vi "0805_Visão_de_máquina.vi"() -> ()   [LabVIEW 2017]
uses:
  <vilib>/userdefined/High Color/IMAQdx.ctl
  <vilib>/vision/driver/IMAQdx.llb/IMAQdx Acquisition Mode.ctl
  <vilib>/vision/driver/IMAQdx.llb/IMAQdx Buffer Number Mode.ctl
  <vilib>/vision/Classification.llb/IMAQ Classifier Read Options.ctl
  <vilib>/vision/driver/NI_Vision_Acquisition_Software.lvlib
  <vilib>/vision/NI_Vision_Development_Module.lvlib
panel:
  out "seletou_detectou":bool
  in  "file (use dialog)":path
  in  "Comunicação de dados":bool
  out "concatenated string 2":string
  out "concatenated string":string
  out "Boolean":bool
  out "Parar_esteira":bool
  out "aux":bool
  out "normal":u32
  out "parou":u32
  out "detectou":u32
  out "Detectou":bool
  out "reconheceu":bool
  out "bool_parou":bool
  out "bool_normal":bool
  out "bool_detectou":bool
  out "reconhecendo":bool
  out "Stop 3":bool
  out "seletor":enum16{"normal", "detectou", "parou"}(ring)=enum."detectou"
  in  "enum":enum16{"normal", "detectou", "parou"}(ring)=enum."detectou"
  out "x .and. y?":bool
  in  "dimensão_x_ROI_esteira":sgl=30.0
  in  "dimensão_y_ROI_esteira":sgl=30.0
  in  "posicao_y_ROI_esteira":sgl
  in  "posicao_x_ROI_esteira":sgl
  out "Local destino":T1(ring)
  in  "Tab Control":T2(tab)
  in  "Cluster A":T3
  in  "Cluster B":T3
  in  "Cluster C":T3
  in  "QRCode":bool
  out "Table":string[][](table)
  in  "Stop 2":bool
  in  "Stop 1":bool
  out "Imagem Original":T4(plugin-control)
  in  "Câmera":T5="cam1"
  out "XY Graph 2":cluster{"X":dbl, "Y":dbl}[](graph)
  # "ROTINA DE VISÃO COMPUTACIONAL"
  # "HISTÓRICO DE RECONHECIMENTO"
  # "DEFINI敲O DA ROI DA ESTEIRA"
  # "IMAGEM OBTIDA PELA CÂMERA"
  # "POSI敲O X"
  # "-100"
  # "POSI敲O Y"
  # "-230"
  # "DIMENSÃO X"
  # "80"
  # "DIMENSÃO Y"
  # "250"
  # "DEFINI敲O DOS LOCAIS DE DESTINO\nDA MANIPULA敲O"
  # "LOCAL DE DESTINO"
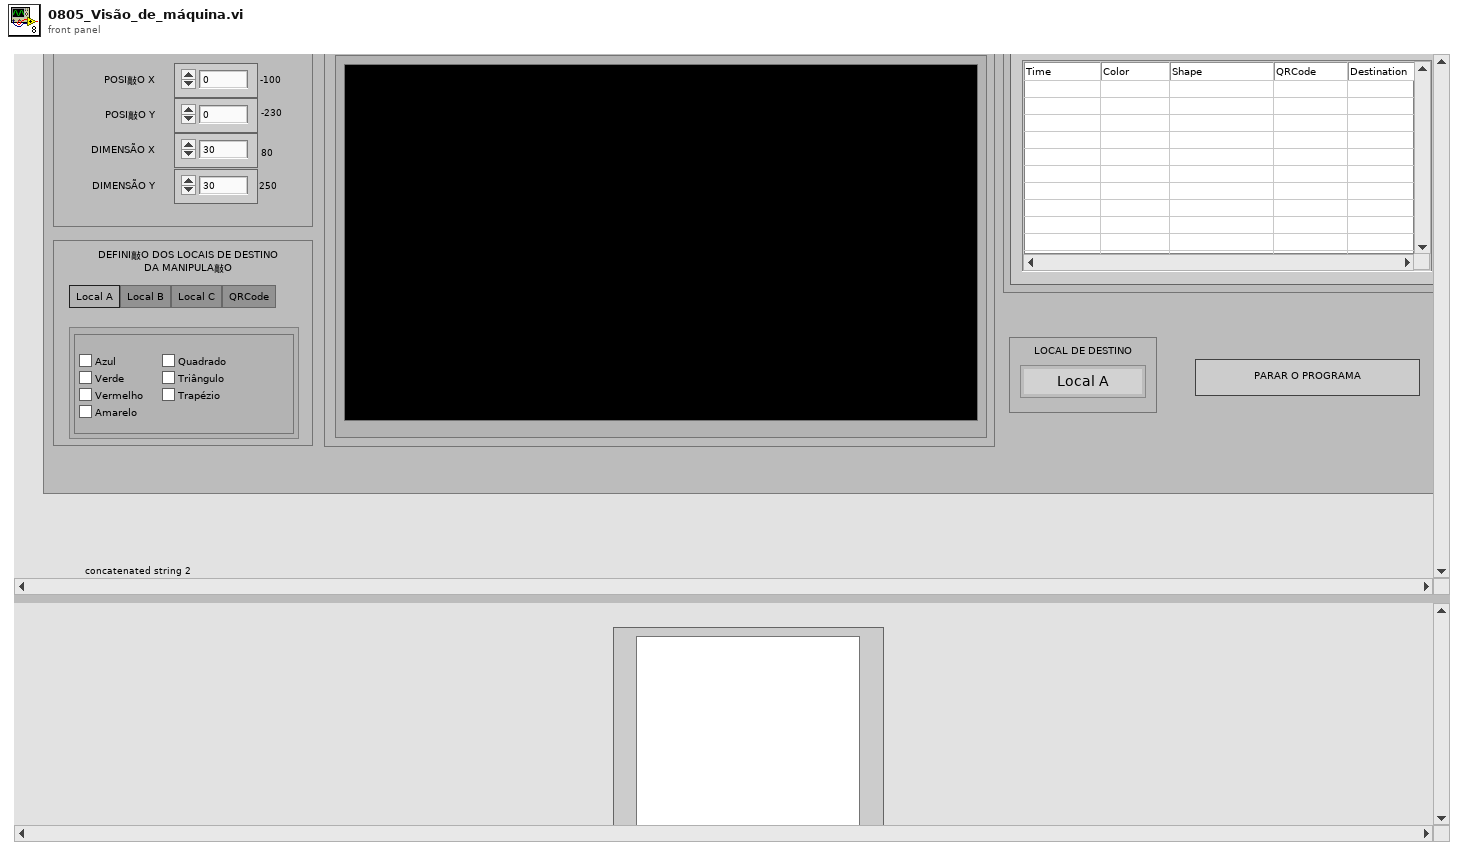
[diagram p1: front panel]
types:
  T1 = enum16{"Local A", "Local B", "Local C", "Discard"}
  T2 = enum32{"Local A", "Local B", "Local C", "QRCode"}
  T3 = cluster{"Azul":bool, "Verde":bool, "Vermelho":bool, "Amarelo":bool, "Quadrado":bool, "Triângulo":bool, "Trapézio":bool}
  T4 = typedef "IMAQ Image.ctl" = refnum<image>
  T5 = typedef "IMAQdx.ctl" = refnum<k21>
  T6 = typedef "NI_Vision_Acquisition_Software.lvlib/IMAQdx Acquisition Mode.ctl" = enum32{"One Shot", "Continuous"}
  T7 = typedef "NI_Vision_Acquisition_Software.lvlib/IMAQdx Buffer Number Mode.ctl" = enum32{"Next", "Last", "Buffer Number", "Every", "Last New"}
  T8 = cluster{"Global Rectangle":i32[], "Contours":cluster{"Contour Type":u32, "ROI Type":u32, "Points":i32[]}[]}
  T9 = typedef "ROI Descriptor" = cluster{"Global Rectangle":i32[], "Contours":cluster{"ID":enum32{"External", "Internal"}, "Type":u32, "Coordinates":i32[]}[]}
  T10 = typedef "IMAQ Classifier Read Options.ctl" = i32
  T11 = typedef "IMAQ Classifier Session.ctl" = refnum<k1>
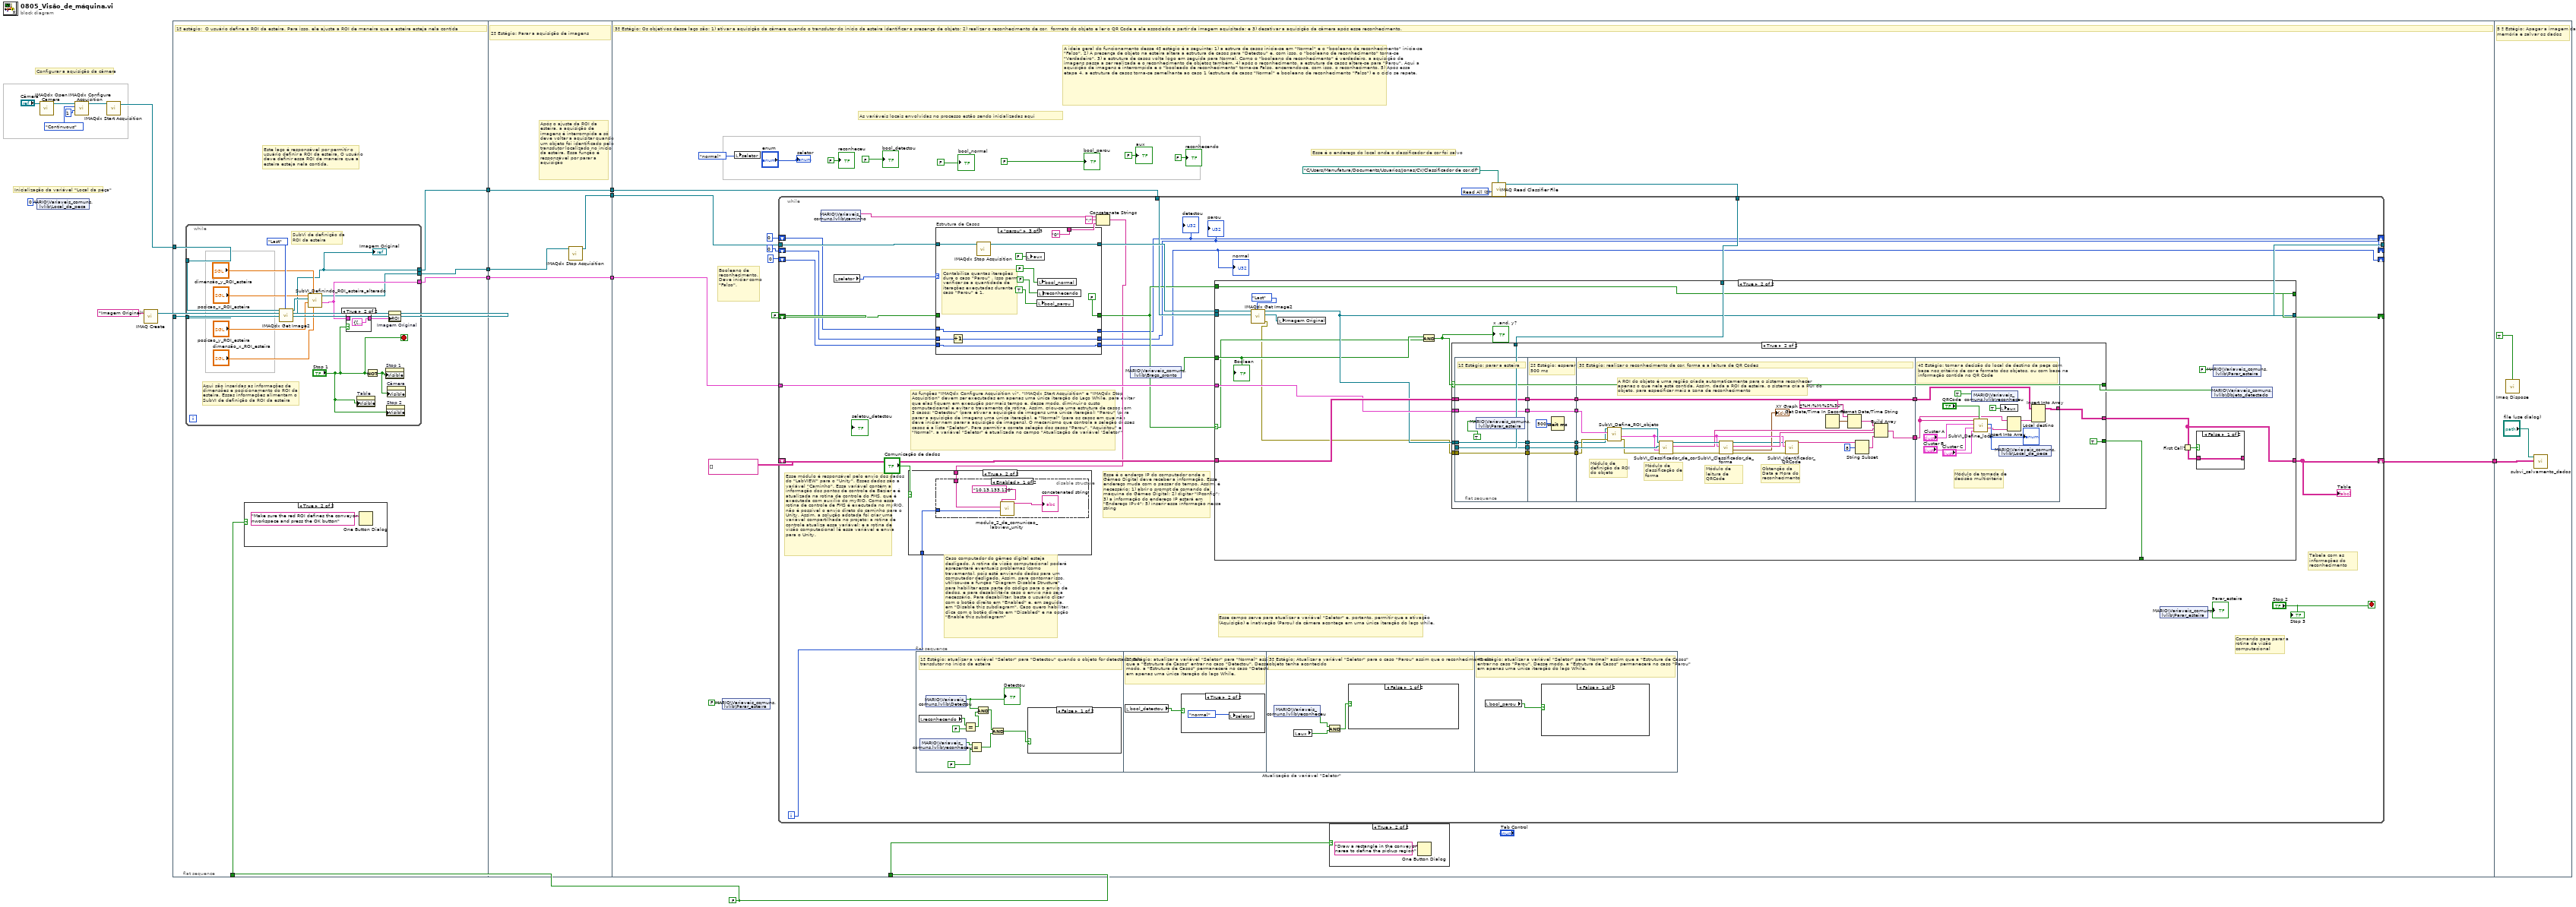
[diagram p0: block diagram]
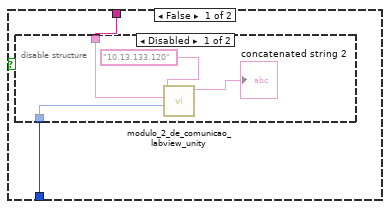
[diagram p4: hidden frame]
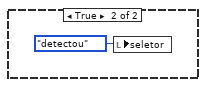
[diagram p7: hidden frame]
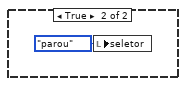
[diagram p9: hidden frame]
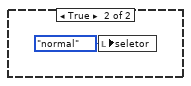
[diagram p10: hidden frame]
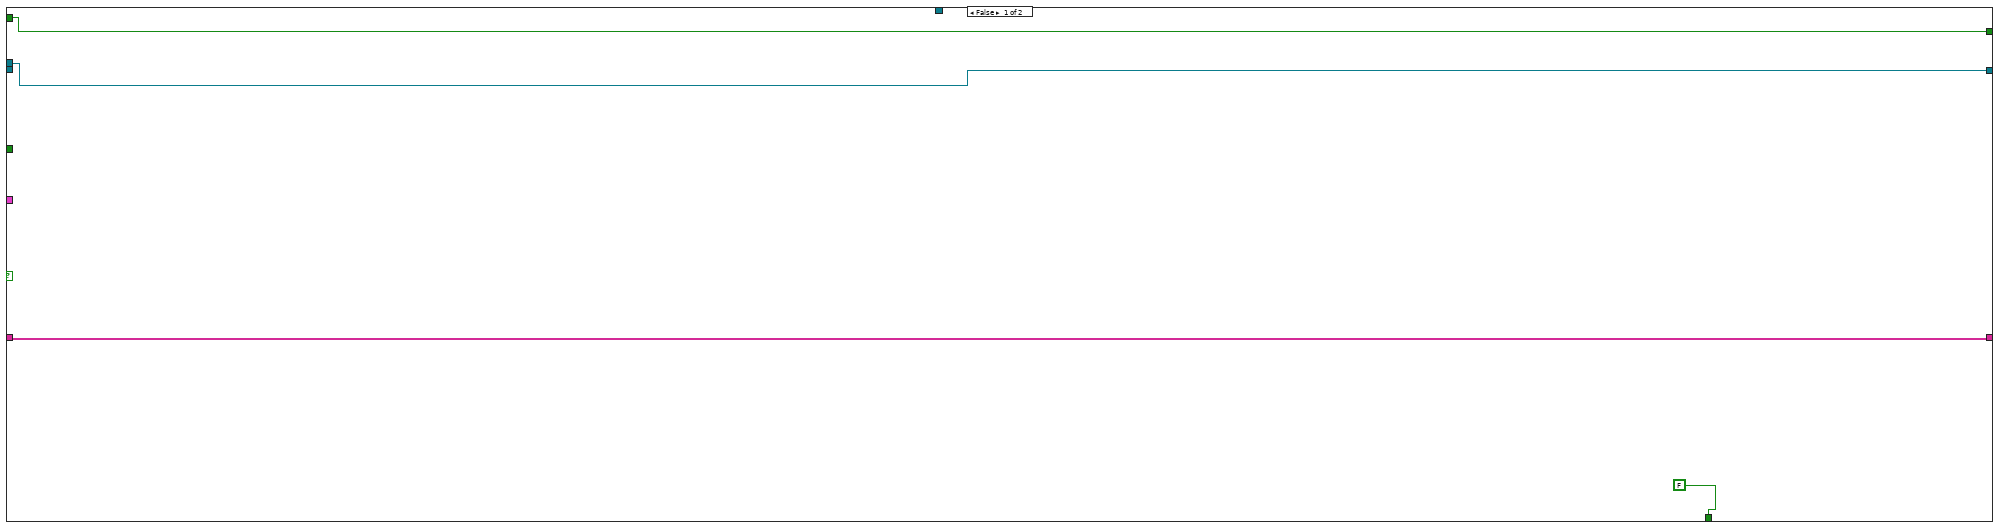
[diagram p11: hidden frame]
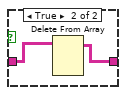
[diagram p12: hidden frame]
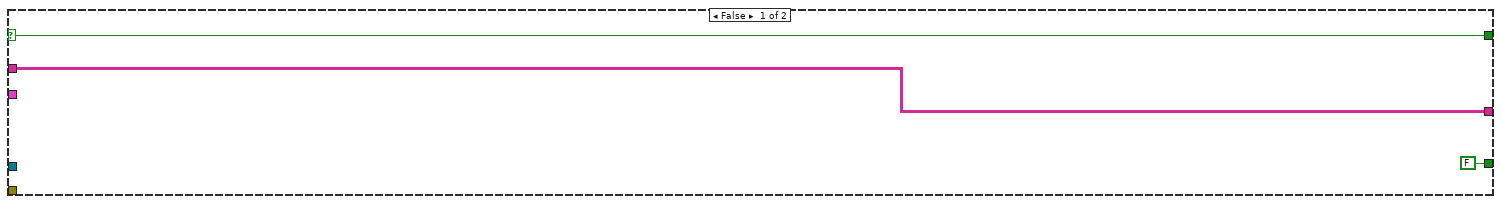
[diagram p13: hidden frame]
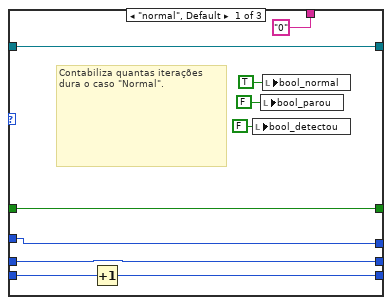
[diagram p14: hidden frame]
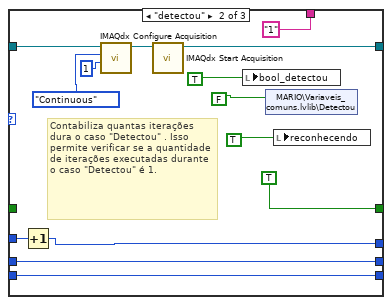
[diagram p15: hidden frame]
diagram:
  w10 = FALSE
  # "Inicialização da variável \"Local da peça\""
  # "Configurar a aquisição da câmera"
  n1 = shared-variable "MARIO\\Variaveis_comuns.lvlib\\Local_da_peca"(i8 0 ("Local_da_peca")) -> ()  [unwired: 1 in, 1 out]
  n2 = call <vilib>:"IMAQdx Open Camera.vi"("Session In"="Câmera") -> ("Session Out"=w17:T5)  [unwired: 9 in, 1 out]
  n3 = call <vilib>:"IMAQdx Configure Acquisition.vi"("Number of Buffers"=u32 1, "Continuous?"=IMAQdx_Acquisition_Mode."Continuous", "Session In"=w17) -> ("Session Out"=w16:T5)  [unwired: 7 in, 1 out]
  n4 = call <vilib>:"IMAQdx Start Acquisition.vi"("Session In"=w16) -> ("Session Out"=w7:T5)  [unwired: 9 in, 1 out]
  n5 = call "IMAQ Create"("Image Name"="Imagem Original") -> ("New Image"=w11:T4)  [unwired: 4 in, 1 out]
  n6 = flat-sequence {
    tunnel: w7 -> [w23]
    tunnel: w11 -> [w22]
    tunnel: [w21] -> w4
    tunnel: [w20] -> w3
    tunnel: [w19] -> w2
    tunnel: w10 -> [w18]
    tunnel: w4 -> [w43]
    tunnel: w3 -> [w44]
    tunnel: [w44] -> w9
    tunnel: [w42] -> w8
    tunnel: w2 -> [w42]
    tunnel: [w41] -> w6
    tunnel: w9 -> [w62]
    tunnel: w10 -> [w66]
    tunnel: w8 -> [w59]
    tunnel: w6 -> [w57]
    tunnel: [w45] -> w1
    tunnel: w1 -> [w256]
    frame #0 {
      # "Este laço é responsável por permitir o usuário definir a ROI da esteira. O usuário deve definir essa ROI de maneira que a esteira esteja nela contida."
      # "1º estágio:  O usuário define a ROI da esteira. Para isso, ele ajusta a ROI de maneira que a esteira esteja nela contida"
      n7 = while {
        tunnel: w23 -> [w37]
        tunnel: w22 -> [w36]
        tunnel: [w26] -> w21
        tunnel: [w27] -> w20
        tunnel: [w25] -> w19
        stop <- "Stop 1" stop-if-true
        # "SubVi de definição da ROI da esteira"
        # "Aqui são inseridas as informações de dimensões e posicionamento do ROI da esteira. Essas informações alimentam o SubVI de definição da ROI da esteira"
        n8 = call <vilib>:"IMAQdx Get Image2.vi"("Buffer Number Mode (Next)"=IMAQdx_Buffer_Number_Mode."Last", "Image In"=w36, "Session In"=w37) -> ("Image Out"=w25:T4, "Session Out"=w28:T5)  [unwired: 5 in, 2 out]
        "Imagem Original" <- w25
        n9 = call "SubVI_Definindo_ROI_esteira_alterado.vi"("largura_y"="dimensão_x_ROI_esteira", "largura_x"="dimensão_y_ROI_esteira", "ofset y"="posicao_y_ROI_esteira", "Session in"=w28, "ofset x"="posicao_x_ROI_esteira") -> ("ROI Descriptor"=w27:T9, "Session Out"=w26:T5)  [unwired: 4 in, 1 out]
        n10 = case shown="True" "Stop 1" {
          tunnel: w27 -> [w39 _]
          tunnel: [w39 T8 {"Global Rectangle"=[0, 0, 1, 1], "Contours"=[{"Contour Type"=0, "ROI Type"=1, "Points"=[0, 0]}]} ("ROI")] -> w35
          frame False {
          }
          frame True {
          }
        }
        n11 = property on="Table" class="Tbl (strict)"("Visible"="Stop 1") -> ()  [unwired: 2 in, 2 out]
        n12 = Not(x="Stop 1") -> (.not. x?=w34:bool)
        n13 = property on="Stop 1" class="Bool"("Visible"=w34) -> ()  [unwired: 2 in, 2 out]
        n14 = property on="Stop 2" class="Bool"("Visible"="Stop 1") -> ()  [unwired: 2 in, 2 out]
        n15 = property on="Câmera" class="IMAQdx (strict)"("Visible"=w34) -> ()  [unwired: 2 in, 2 out]
        n16 = property on="Imagem Original" class="ImageControl"("ROI"=w35) -> ()  [unwired: 2 in, 2 out]
      }
      n17 = case shown="True" w18 {
        frame False {
        }
        frame True {
          n18 = One Button Dialog(message="Make sure the red ROI defines the conveyor \nworkspace and press the OK button") -> ()  [unwired: 1 in, 1 out]
        }
      }
    }
    frame #1 {
      # "Após o ajuste da ROI da esteira, a aquisição de imagens é interrompida e só deve voltar a aquisitar quando um objeto foi identificado pelo transdutor localizado no início da esteira. Essa função é responsável por parar a aquisição"
      # "2º Estágio: Parar a aquisição de imagens"
      n19 = call <vilib>:"IMAQdx Stop Acquisition.vi"("Session In"=w43) -> ("Session Out"=w41:T5)  [unwired: 9 in, 1 out]
    }
    frame #2 {
      w65 = T10 0 items=["Read All", "Add Samples, Do Not Change Options", "Read Options, Do Not Add Samples"] ("Read Options")
      # "Esse é o endereço do local onde o classificador de cor foi salvo"
      # "A ideia geral do funcionamento desse 4º estágio é a seguinte: 1) a estrura de casos inicia-se em \"Normal\" e o \"booleano de reconhecimento\" inicia-se \"Falso\". 2) A presença de objeto na esteira altera a estrutura de casos para \"Detectou\" e, com isso, o \"booleano de reconhecimento\" torna-se \"Verdadeiro\". 3) a estrutura de casos volta logo em seguida para Normal. Como o \"booleano de reconhecimento\" é verdadeiro, a aquisição de imagens passa a ser realizada e o reconhecimento de objetos também. 4) após o reconhecimento, a estrutura de casos altera-se para \"Parou\". Aqui a aquisição de imagens é interrompida e o \"booleado de reconhecimento\" torna-se Falso, encerrando-se, com isso, o reconhecimento. 5) Após essa etapa 4, a estrutura de casos torna-se semelhante ao caso 1 (estrutura de casos \"Normal\" e booleano de reconhecimento \"Falso\") e o ciclo se repete."
      # "As variáveis locais envolvidas no processo estão sendo inicializadas aqui"
      # "Booleano de reconhecimento. Deve iniciar como \"Falso\"."
      # "3º Estágio: Os objetivos desse laço são: 1) ativar a aquisição da câmera quando o transdutor do início da esteira identificar a presença de objeto; 2) realizar o reconhecimento de cor,  formato do objeto e ler o QR Code a ele associado a partir da imagem aquisitada; e 3) desativar a aquisição da câmera após esse reconhecimento."
      n20 = shared-variable "MARIO\\Variaveis_comuns.lvlib\\Parar_esteira"(FALSE ("Parar_esteira")) -> ()  [unwired: 1 in, 1 out]
      n21 = local write "seletor"(enum16{"normal", "detectou", "parou"}."normal") -> ()
      n22 = case shown="True" w66 {
        frame False {
        }
        frame True {
          n23 = One Button Dialog(message="Draw a rectangle in the conveyor\narea to define the pickup region") -> ()  [unwired: 1 in, 1 out]
        }
      }
      n24 = call "IMAQ Read Classifier File"("File Path"=path "C:/Users/Manufatura/Documents/Usuarios/Jonas/CV/Classificador de cor.clf", "Read Options"=w65) -> ("Classifier Session"=w64:T11)  [unwired: 2 in, 7 out]
      n25 = while {
        tunnel: w62 -> [w92]
        tunnel: w64 -> [w93]
        shift-right: [w73] -> w45
        shift-left: string[][] [] ("Table") -> [w74]
        tunnel: w59 -> [w90]
        shift-right: [w87] -> _
        shift-left: FALSE -> [w89]
        tunnel: w57 -> [w85]
        tunnel: [w86] -> _
        shift-right: [w81] -> _
        shift-left: u32 0 ("Number of Buffers") -> [w78]
        shift-right: [w80] -> _
        shift-left: u32 0 ("Number of Buffers") -> [w77]
        shift-right: [w79] -> _
        shift-left: u32 0 ("Number of Buffers") -> [w76]
        i -> [w68]
        stop <- "Stop 2" stop-if-true
        # "Tabela com as informações do reconhecimento"
        # "Comando para parar a rotina de visão computacional"
        # "Esse campo serve para atualizar a variável \"Seletor\" e, portanto, permitir que a ativação (Aquisição) e inativação (Parou) da câmera aconteça em uma única iteração do laço while."
        # "Esse é o enderço IP do computador onde o Gêmeo Digital deve receber a informação. Esse endereço muda com o passar do tempo. Assim, é necessário: 1) abrir o prompt de comando da máquina do Gêmeo Digital; 2) digitar \"IPconfig\"; 3) a informação do endereço IP estará em \"Endereço IPv4\"; 5) inserir essa informação nessa string"
        # "Caso computador do gêmeo digital esteja desligado, A rotina de visão computacional poderá apresentará eventuais problemas (como travamento), pois está enviando dados para um computador desligado. Assim, para contornar isso, utilizou-se a função \"Diagram Disable Structure\", para habilitar essa parte do código para o envio de dados, e para desabilitá-la caso o envio não seja necessário. Para desabilitar, basta o usuário clicar com o botão direito em \"Enabled\" e, em seguida, em \"Disable this subdiagram\". Caso quero habilitar, clica com o botão direito em \"Disabled\" e na opção \"Enable this subdiagram\""
        # "Esse módulo é responsável pelo envio dos dados do \"LabVIEW\" para o \"Unity\". Esses dados são a variável \"Caminho\". Essa variável contém a informação dos pontos de controle de Bézier e é atualizada na rotina de controle do FMS, que é executada com auxílio do myRIO. Como essa rotina de controle de FMS é executada no myRIO, não é possível o envio direto do caminho para o Unity. Assim, a solução adotada foi criar uma  variável compartilhada no projeto: a rotina de controle atualiza essa variável; e a rotina de visão computacional lê essa variável e envia para o Unity."
        # "As funções \"IMAQdx Configure Acquisition vi\", \"IMAQdx Start Acquisition\" e \"IMAQdx Stop Acquisition\" devem ser executadas em apenas uma única iteração do Laço While, para evitar que elas fiquem em execução por mais tempo e, desse modo, diminuir o custo computacioanal e evitar o travamento da rotina. Assim, criou-se uma estrutura de casos com 3 casos: \"Detectou\" (para ativar a aquisição de imagens uma única iteração); \"Parou\" (para parar a aquisição de imagens uma única iteração), e \"Normal\" (para os casos em que não deve iniciar nem parar a aquisição de imagens). O mecanismo que controla a seleção desses casos é a lista \"Seletor\". Para permitir a correta seleção dos casos \"Parou\", \"Aquisitou\" e \"Normal\", a variável \"Seletor\" é atualizada no campo \"Atualização da variável 'Seletor'\""
        n26 = shared-variable "MARIO\\Variaveis_comuns.lvlib\\caminho"() -> (w71:string)  [unwired: 1 in, 1 out]
        n27 = local read "seletor"() -> (w82:enum16{"normal", "detectou", "parou"})
        n28 = flat-sequence "Atualização da variável \"Seletor\"" {
          frame #0 {
            # "1º Estágio: atualizar a variável \"Seletor\" para \"Detectou\" quando o objeto for detectado pelo transdutor no início da esteira"
            n29 = local read "reconhecendo"() -> (w110:bool)
            n30 = shared-variable "MARIO\\Variaveis_comuns.lvlib\\reconheceu"() -> (w112:bool)  [unwired: 1 in, 1 out]
            n31 = shared-variable "MARIO\\Variaveis_comuns.lvlib\\Detectou"() -> (w108:bool)  [unwired: 1 in, 1 out]
            "Detectou" <- w108
            n32 = Equal?(x=w110, y=FALSE) -> (x = y?=w111:bool)
            n33 = Equal?(x=w112, y=FALSE) -> (x = y?=w113:bool)
            n34 = And(x=w108, y=w111) -> (x .and. y?=w109:bool)
            n35 = And(x=w109, y=w113) -> (x .and. y?=w114:bool)
            n36 = case shown="False" w114 {
              frame False {
              }
              frame True {
                n37 = local write "seletor"(enum16{"normal", "detectou", "parou"}."detectou") -> ()
              }
            }
          }
          frame #1 {
            # "2º Estágio: atualizar a variável \"Seletor\" para \"Normal\" assim que a \"Estrutura de Casos\" entrar no caso \"Detectou\". Desse modo, a \"Estrutura de Casos\" permanecerá no caso \"Detectou\" em apenas uma única iteração do laço While."
            n38 = local read "bool_detectou"() -> (w116:bool)
            n39 = case shown="True" w116 {
              frame False {
              }
              frame True {
                n40 = local write "seletor"(enum16{"normal", "detectou", "parou"}."normal") -> ()
              }
            }
          }
          frame #2 {
            # "3º Estágio: Atualizar a variável \"Seletor\" para o caso \"Parou\" assim que o reconhecimento do objeto tenha acontecido"
            n41 = shared-variable "MARIO\\Variaveis_comuns.lvlib\\reconheceu"() -> (w120:bool)  [unwired: 1 in, 1 out]
            n42 = local read "aux"() -> (w119:bool)
            n43 = And(x=w120, y=w119) -> (x .and. y?=w118:bool)
            n44 = case shown="False" w118 {
              frame False {
              }
              frame True {
                n45 = local write "seletor"(enum16{"normal", "detectou", "parou"}."parou" ("lista")) -> ()
              }
            }
          }
          frame #3 {
            # "4º estágio: atualizar a variável \"Seletor\" para \"Normal\" assim que a \"Estrutura de Casos\" entrar no caso \"Parou\". Desse modo, a \"Estrutura de Casos\" permanecerá no caso \"Parou\" em apenas uma única iteração do laço While."
            n46 = local read "bool_parou"() -> (w122:bool)
            n47 = case shown="False" w122 {
              frame False {
              }
              frame True {
                n48 = local write "seletor"(enum16{"normal", "detectou", "parou"}."normal" ("lista")) -> ()
              }
            }
          }
        }
        n49 = case "Estrutura de Casos" shown="\"parou\"" w82 {
          tunnel: [w226 w237 w252] -> w91
          tunnel: w85 -> [w226 w238 w253]
          tunnel: [w227 TRUE FALSE] -> w88
          tunnel: w89 -> [w227 _ _]
          tunnel: w78 -> [w221 w232 w245]
          tunnel: w77 -> [w220 w230 w247]
          tunnel: w76 -> [w222 w229 w244]
          tunnel: [w221 w231 w245] -> w81
          tunnel: [w220 w230 w246] -> w80
          tunnel: [w219 w229 w244] -> w79
          tunnel: ["0" ("string") "1" ("string") "0" ("string")] -> w69
          frame "normal", Default {
            # "Contabiliza quantas iterações dura o caso \"Normal\"."
            n50 = Increment(x=w222) -> (x+1=w219:u32)
            n51 = local write "bool_detectou"(FALSE ("detectou")) -> ()
            n52 = local write "bool_parou"(FALSE ("bool_parou")) -> ()
            n53 = local write "bool_normal"(TRUE ("bool_normal")) -> ()
          }
          frame "detectou" {
            # "Contabiliza quantas iterações dura o caso \"Detectou\" . Isso permite verificar se a quantidade de iterações executadas durante o caso \"Detectou\" é 1."
            n54 = Increment(x=w232) -> (x+1=w231:u32)
            n55 = call <vilib>:"IMAQdx Configure Acquisition.vi"("Number of Buffers"=u32 1, "Continuous?"=IMAQdx_Acquisition_Mode."Continuous", "Session In"=w238) -> ("Session Out"=w239:T5)  [unwired: 7 in, 1 out]
            n56 = call <vilib>:"IMAQdx Start Acquisition.vi"("Session In"=w239) -> ("Session Out"=w237:T5)  [unwired: 9 in, 1 out]
            n57 = local write "bool_detectou"(TRUE ("bool_detectou")) -> ()
            n58 = shared-variable "MARIO\\Variaveis_comuns.lvlib\\Detectou"(FALSE ("Detectou")) -> ()  [unwired: 1 in, 1 out]
            n59 = local write "reconhecendo"(TRUE ("reconhecendo")) -> ()
          }
          frame "parou" {
            # "Contabiliza quantas iterações dura o caso \"Parou\" . Isso permite verificar se a quantidade de iterações executadas durante o caso \"Parou\" é 1."
            n60 = Increment(x=w247) -> (x+1=w246:u32)
            n61 = call <vilib>:"IMAQdx Stop Acquisition.vi"("Session In"=w253) -> ("Session Out"=w252:T5)  [unwired: 9 in, 1 out]
            n62 = local write "aux"(FALSE ("aux")) -> ()
            n63 = local write "bool_parou"(TRUE ("bool_parou")) -> ()
            n64 = local write "bool_normal"(FALSE ("bool_normal")) -> ()
            n65 = local write "reconhecendo"(FALSE ("reconhecendo")) -> ()
          }
        }
        "detectou" <- w81
        "parou" <- w80
        "normal" <- w79
        n66 = Concatenate Strings(w71, ";" ("string"), w69) -> (w67:string)
        n67 = case shown="True" "Comunicação de dados" {
          tunnel: w68 -> [w95 w101]
          tunnel: w67 -> [w94 w100]
          frame False {
            n68 = disable-structure shown="Disabled" {
              disable-tunnel: w95 -> [w97 _]
              disable-tunnel: w94 -> [w96 _]
              frame Disabled {
                n69 = call "modulo_2_de_comunicao_labview_unity.vi"("number"=w97, "String"=w96, "address"="10.13.133.120") -> ("concatenated string"=→"concatenated string 2":string)  [unwired: 7 in, 1 out]
              }
              frame Enabled {
              }
            }
          }
          frame True {
            n70 = disable-structure shown="Enabled" {
              disable-tunnel: w101 -> [w103 _]
              disable-tunnel: w100 -> [w102 _]
              frame Enabled {
                n71 = call "modulo_2_de_comunicao_labview_unity.vi"("number"=w103, "String"=w102, "address"="10.13.133.120") -> ("concatenated string"=→"concatenated string":string)  [unwired: 7 in, 1 out]
              }
              frame Disabled {
              }
            }
          }
        }
        n72 = shared-variable "MARIO\\Variaveis_comuns.lvlib\\Braço_pronto"() -> (w84:bool)  [unwired: 1 in, 1 out]
        n73 = case shown="True" w88 {
          selector: w88 -> [_ w132]
          tunnel: w93 -> [_ w145]
          tunnel: w74 -> [w127 w144]
          tunnel: [w127 w128] -> w73
          tunnel: w92 -> [_ w141]
          tunnel: w91 -> [w125 w138]
          tunnel: w90 -> [_ w137]
          tunnel: [w126 w135] -> w87
          tunnel: w88 -> [w126 w135]
          tunnel: [w125 w136] -> w86
          tunnel: w84 -> [_ w133]
          tunnel: [FALSE w134] -> _
          frame False {
          }
          frame True {
            n74 = call <vilib>:"IMAQdx Get Image2.vi"("Buffer Number Mode (Next)"=IMAQdx_Buffer_Number_Mode."Last", "Image In"=w137, "Session In"=w138) -> ("error out"=w129:errorcluster, "Image Out"=w139:T4, "Session Out"=w136:T5)  [unwired: 5 in, 1 out]
            n75 = local write "Imagem Original"(w139) -> ()
            n76 = And(x=w133, y=w132) -> (x .and. y?=w131:bool)
            "x .and. y?" <- w131
            n77 = case shown="True" w131 {
              selector: w131 -> [w150 w165]
              tunnel: w136 -> [_ w169]
              tunnel: w145 -> [_ w171]
              tunnel: w129 -> [_ w170]
              tunnel: [w151 w168] -> w128
              tunnel: w144 -> [w151 w167]
              tunnel: [w150 w165] -> w142
              tunnel: w141 -> [_ w164]
              tunnel: [FALSE TRUE] -> w134
              frame False {
              }
              frame True {
                n78 = flat-sequence {
                  tunnel: w167 -> [w174]
                  tunnel: w169 -> [w175]
                  tunnel: w170 -> [w176]
                  tunnel: w171 -> [w177]
                  tunnel: [w177] -> w163
                  tunnel: [w176] -> w161
                  tunnel: [w175] -> w159
                  tunnel: [w174] -> w157
                  tunnel: w164 -> [w173]
                  tunnel: [w173] -> w155
                  tunnel: w163 -> [w183]
                  tunnel: [w183] -> w162
                  tunnel: w161 -> [w182]
                  tunnel: [w182] -> w160
                  tunnel: w159 -> [w181]
                  tunnel: [w181] -> w158
                  tunnel: w157 -> [w180]
                  tunnel: [w180] -> w156
                  tunnel: w155 -> [w179]
                  tunnel: [w179] -> w154
                  tunnel: [w194] -> w166
                  tunnel: w162 -> [w205]
                  tunnel: w160 -> [w191]
                  tunnel: w158 -> [w189]
                  tunnel: w156 -> [w186]
                  tunnel: w154 -> [w192]
                  tunnel: [w186] -> w153
                  tunnel: w166 -> [w210]
                  tunnel: w153 -> [w212]
                  tunnel: [w211] -> w168
                  frame #0 {
                    # "1º Estágio: parar a esteira"
                    n79 = shared-variable "MARIO\\Variaveis_comuns.lvlib\\Parar_esteira"(TRUE ("Parar_esteira")) -> ()  [unwired: 1 in, 1 out]
                  }
                  frame #1 {
                    # "2º Estágio: esperar 500 ms"
                    n80 = Wait (ms)(milliseconds to wait=u32 500) -> ()  [unwired: 1 out]
                  }
                  frame #2 {
                    # "A ROI do objeto é uma região criada automaticamente para o sistema reconhecer apenas o que nela está contida. Assim, dada a ROI da esteira, o sistema cria a ROI do objeto, para especificar mais a zona de reconhecimento"
                    # "Módulo de definição da ROI do objeto"
                    # "Módulo de classificação de forma"
                    # "Módulo de leitura de QRCode"
                    # "Obtenção da Data e Hora do reconhecimento"
                    # "3º Estágio: realizar o reconhecimento de cor, forma e a leitura de QR Codes"
                    n81 = call "SubVI_Define_ROI_objeto.vi"("error in (no error)"=w191, "ROI Esteira"=w192, "Session In"=w189) -> ("error out"=w190:errorcluster, "ROI Objeto"=w187:T9, "Session Out"=w188:T5)  [unwired: 5 in, 1 out]
                    n82 = call "SubVI_Classificador_de_cor.vi"("error in"=w190, "ROI Objeto"=w187, "Classifier Session"=w205, "Session In"=w188) -> ("error out"=w204:errorcluster, "Class"=w193:string, "Session Out"=w199:T5)  [unwired: 5 in]
                    n83 = call "SubVI_Classificador_de_forma.vi"("error in"=w204, "ROI Objeto"=w187, "Session In"=w199) -> ("error out"=w200:errorcluster, "Points"=→"XY Graph 2":cluster{"X":dbl, "Y":dbl}[], "Forma"=w198:string, "Session Out"=w184:T5)  [unwired: 5 in]
                    n84 = call "SubVI_Identificador_QRCode.vi"("error in"=w200, "ROI Objeto"=w187, "Session In"=w184) -> ("Data"=w197:string)  [unwired: 7 in, 1 out]
                    n85 = Get Date/Time In Seconds() -> (seconds since 1Jan1904=w202:timestamp)
                    n86 = Format Date/Time String(time format string (%c)="%H:%M:%S%3u", seconds (now)=w202) -> (date/time string=w201:string)  [unwired: 1 in]
                    n87 = String Subset(string=w197, offset (0)=8) -> (substring=w196:string)  [unwired: 1 in]
                    n88 = Build Array(w201, w193, w198, w196) -> (w194:string[])
                  }
                  frame #3 {
                    # "Módulo de tomada de decisão multicritério"
                    # "4º Estágio: tomar a decisão do local de destino da peça com base nos critéirio de cor e formato dos objetos, ou com base na informação contida no QR Code"
                    n89 = shared-variable "MARIO\\Variaveis_comuns.lvlib\\reconheceu"(TRUE ("reconheceu")) -> ()  [unwired: 1 in, 1 out]
                    n90 = call "SubVI_Define_local.vi"("QRCode"="QRCode", "Cluster C"="Cluster C", "Cluster B"="Cluster B", "Cluster A"="Cluster A", "Linha da tabela"=w210) -> ("Destino"=w208:string, "Local destino"=w214:T1)  [unwired: 5 in]
                    "Local destino" <- w214
                    n91 = shared-variable "MARIO\\Variaveis_comuns.lvlib\\Local_da_peca"(w214) -> ()  [unwired: 1 in, 1 out]
                    n92 = local write "aux"(TRUE ("aux")) -> ()
                    n93 = Insert Into Array(array=w210, new element=w208) -> (w209:string[])  [unwired: 1 in]
                    n94 = Insert Into Array(array=w212, new element=w209) -> (w211:string[][])  [unwired: 2 in]
                  }
                }
              }
            }
            n95 = First Call?() -> (First Call?: T/F=w143:bool)
            n96 = case shown="False" w143 {
              tunnel: w128 -> [w146 w148]
              tunnel: [w146 w147] -> _
              frame False {
              }
              frame True {
                n97 = Delete From Array(array=w148) -> (array with subset deleted=w147:string[][])  [unwired: 3 in, 1 out]
              }
            }
            n98 = shared-variable "MARIO\\Variaveis_comuns.lvlib\\Objeto_detectado"(w142) -> ()  [unwired: 1 in, 1 out]
            n99 = shared-variable "MARIO\\Variaveis_comuns.lvlib\\Parar_esteira"(FALSE ("Parar_esteira")) -> ()  [unwired: 1 in, 1 out]
            "Boolean" <- w133
          }
        }
        "Table" <- w73
        n100 = shared-variable "MARIO\\Variaveis_comuns.lvlib\\Parar_esteira"() -> (→"Parar_esteira":bool)  [unwired: 1 in, 1 out]
        "Stop 3" <- "Stop 2"
      }
      "reconhecendo" <- FALSE ("reconheceu")
      "seletor" <- "enum"
      "bool_detectou" <- FALSE
      "bool_normal" <- FALSE
      "bool_parou" <- FALSE
      "reconheceu" <- FALSE ("reconheceu")
      "aux" <- FALSE
    }
    frame #3 {
      # "5 º Estágio: Apagar a imagem da memória e salvar os dados"
      n101 = call "Imaq Dispose"("All Images? (No)"=TRUE) -> ()  [unwired: 5 in, 1 out]
      n102 = call "subvi_salvamento_dados.vi"("Table"=w256, "file (use dialog)"="file (use dialog)") -> ()  [unwired: 9 in, 1 out]
    }
  }
